vi "Bug2 PlanMod.vi"() -> ()   [LabVIEW 2013, in "RVCLibrary_Bug2.lvclass"]
uses:
  RVCLibrary_Bug2.lvclass
  <vilib>/robotics/Navigation/Anytime D Star/NI_Robotics_AnytimeDStar.lvclass
  <vilib>/robotics/Navigation/shared/MapNode/AbstractDstarNode/NI_Robotics_AbstractDstarNode.lvclass
panel:
  out "no valid path exists":bool
  out "path references":refnum<data-value>[](array[refnum])
  out "path cost":dbl
  in  "overhaul (F)":bool
  in  "epsilon":dbl=1.0
  in  "new goal reference":refnum<data-value>
  in  "current reference":refnum<data-value>
  out "RVCLibrary_Bug2 out":refnum<class "RVCLibrary_Bug2.lvclass">
  in  "RVCLibrary_Bug2 in":refnum<class "RVCLibrary_Bug2.lvclass">
  out "error out":errorcluster
  in  "error in (no error)":errorcluster
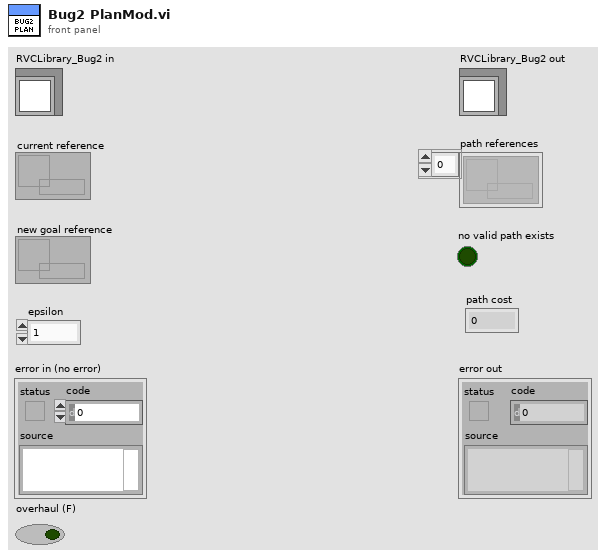
[diagram p1: front panel]
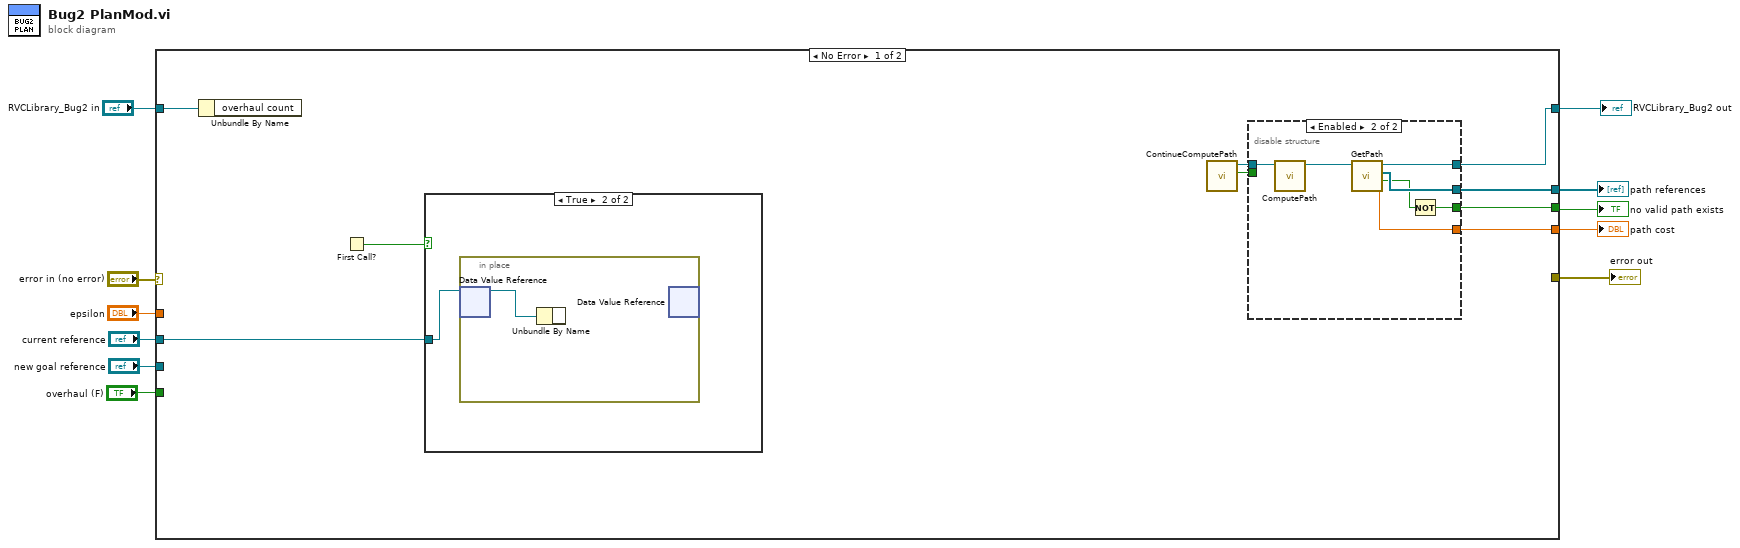
[diagram p0: block diagram]
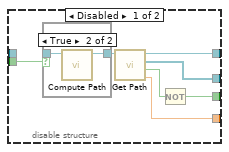
[diagram p3: hidden frame]
diagram:
  n1 = case shown="No Error" "error in (no error)" {
    selector: "error in (no error)" -> [_ w41]
    tunnel: [_ w41] -> w10
    tunnel: [w19 w40] -> w9
    tunnel: "RVCLibrary_Bug2 in" -> [w18 w40]
    tunnel: "current reference" -> [w12 _]
    tunnel: "new goal reference" -> [_ _]
    tunnel: "epsilon" -> [_ _]
    tunnel: "overhaul (F)" -> [_ _]
    tunnel: [w17 _] -> w3
    tunnel: [w16 _] -> w2
    tunnel: [w15 _] -> w1
    frame No Error {
      n2 = Unbundle By Name(w18) -> ()  [unwired: 1 out]
      n3 = First Call?() -> (First Call?: T/F=w13:bool)
      n4 = case shown="True" w13 {
        tunnel: w12 -> [_ w21]
        frame False {
        }
        frame True {
          n5 = in-place {
            n6 = in-place-dvr #1(w21) -> (w22:refnum<class "NI_Robotics_AbstractDstarNode.lvclass">)  [unwired: 1 out]
            n7 = Unbundle By Name(w22) -> ()  [unwired: 1 out]
            n8 = in-place-dvr #1() -> ()  [unwired: 1 in, 2 out]
          }
        }
      }
      n9 = call "ContinueComputePath.vi"() -> ("continue computing path"=w20:bool, "RVCLibrary_Bug2 out"=w14:refnum<class "RVCLibrary_Bug2.lvclass">)  [unwired: 10 in]
      n10 = disable-structure shown="Enabled" {
        disable-tunnel: w20 -> [w29 _]
        disable-tunnel: [w26 w37] -> w19
        disable-tunnel: [w25 w36] -> w17
        disable-tunnel: [w24 w34] -> w16
        disable-tunnel: [w23 w35] -> w15
        disable-tunnel: w14 -> [_ w39]
        frame Disabled {
          n11 = case shown="True" w29 {
            tunnel: [w30 w32] -> w28
            tunnel: _ -> [w30 w31]
            frame False {
            }
            frame True {
              n12 = call <vilib>:"Compute Path.vi"("AD* in"=w31) -> ("AD* out"=w32:refnum<class "NI_Robotics_AnytimeDStar.lvclass">)  [unwired: 10 in]
            }
          }
          n13 = call <vilib>:"Get Path.vi"("AD* in"=w28) -> ("path cost"=w23:dbl, "valid path"=w27:bool, "path"=w25:refnum<data-value>[], "AD* out"=w26:refnum<class "NI_Robotics_AnytimeDStar.lvclass">)  [unwired: 7 in]
          n14 = Not(x=w27) -> (.not. x?=w24:bool)
        }
        frame Enabled {
          n15 = call "ComputePath.vi"("RVCLibrary_Bug2 in"=w39) -> ("RVCLibrary_Bug2 out"=w38:refnum<class "RVCLibrary_Bug2.lvclass">)  [unwired: 10 in]
          n16 = call "GetPath.vi"("RVCLibrary_Bug2 in"=w38) -> ("path cost"=w35:dbl, "valid path"=w33:bool, "path"=w36:refnum<data-value>[], "RVCLibrary_Bug2 out"=w37:refnum<class "RVCLibrary_Bug2.lvclass">)  [unwired: 7 in]
          n17 = Not(x=w33) -> (.not. x?=w34:bool)
        }
      }
    }
    frame Error {
    }
  }
  "error out" <- w10
  "RVCLibrary_Bug2 out" <- w9
  "path cost" <- w1
  "path references" <- w3
  "no valid path exists" <- w2
